vi "rqcBob FPGA.vi"() -> ()   [LabVIEW 2018]
uses:
  rqcBob/Custom Controls/rqcBob Trigger Type.ctl
  rqcBob/Custom Controls/Main State Machine/rqcBob Main SM.ctl
  rqcBob/Custom Controls/Main State Machine/rqcBob Main Operation State.ctl
  rqcBob/Custom Controls/Main State Machine/rqcBob Main Operation Parameters.ctl
  rqcBob/Custom Controls/Pulse Train/rqcBob Pulse Train Config.ctl
  rqcBob/Custom Controls/Pulse Train/rqcBob Pulse Train.Generation Mode.ctl
  rqcBob/Custom Controls/Pulse Train/rqcBob Pulse Train.First Pulse Delay Mode.ctl
  rqcBob/Custom Controls/rqcBob Modulator Config.ctl
  rqcBob/Custom Controls/rqcBob Window Config.ctl
  rqcBob/Custom Controls/rqcBob Detector Settings.ctl
  Shared/Shared FPGA Lib/Shared Logic/Custom Controls/rqc Random Generator.parameters.ctl
  Shared/Shared FPGA Lib/Shared Logic/Custom Controls/rqc Random Generator.value type.ctl
  <vilib>/Platform/TimedLoop/XDataNode/timing_clust.ctl
  <vilib>/Platform/TimedLoop/XDataNode/nitl_modes.ctl
  <vilib>/Platform/TimedLoop/XDataNode/wakeup.ctl
  <vilib>/rvi/Emulation/niFpgaSctlEmulationGetInTimedLoop.vi
  <vilib>/rvi/Emulation/niFpgaEmulationReportErrorSimple.vi
  <vilib>/rvi/Emulation/niFpgaGetClockAttributes.vi
  <vilib>/rvi/Emulation/niFpgaCriticalErrorInLSC.vi
  <vilib>/rvi/eio/common/nirviEmuTemplateMethod_errors.vi
  <vilib>/rvi/Emulation/niFpgaProcessEmulError.vi
  <vilib>/rvi/Emulation/niFpgaEmulationIsFPGAContextNoSignature.vi
  <vilib>/rvi/DataTransferAndStorage/Container/Common/niFpgaContainerGetUniqueNameForEmu.vi
  <vilib>/rvi/Memory/Memory_Emulation/niFpgaMemoryEmulationCacheClearOnFirstRun.vi
  <vilib>/rvi/Memory/Memory_Emulation/nirvimemoryEmulationManagerCache_MakeExclusive.vi
  <vilib>/rvi/Memory/Memory_Emulation/niFpgaMemoryEmulationValidateCache.vi
  <vilib>/rvi/Memory/Memory_Emulation/nirvimemoryEmulationManagerCache_InsertValue.vi
  <vilib>/Utility/error.llb/Clear Errors.vi
  <vilib>/rvi/Memory/Memory_Emulation/nirvimemoryEmulationManagerCache_ReleaseExclusive.vi
  <vilib>/rvi/Memory/Memory_Emulation/nirvimemoryEmulationManagerCache_GetValue.vi
  <vilib>/rvi/Memory/Memory_Emulation/nirvimemoryEmulationManagerCache_SetValue.vi
  <vilib>/rvi/eio/common/nirviEmuReportErrorAndStop.vi
  Shared/Shared FPGA Lib/Shared Logic/FIFO/FIFO.write/rqc FIFO Write (U32).vi
  Shared/Shared FPGA Lib/Shared Logic/FIFO/FIFO.write/rqc FIFO Write (U16).vi
  <vilib>/RQC/FPGA Basic Logic/Counters/Counter (U8).vi
  <vilib>/rvi/DataTransferAndStorage/Container/Common/niFpgaContainerSetEmuInfo.vi
  <vilib>/Platform/TimedLoop/XDataNode/XDataNode.xnode
  <vilib>/eio/EIONode/EIONode.xnode
  <vilib>/rvi/DataTransferAndStorage/Container/XNode/niFpgaContainer.xnode
  <vilib>/rvi/DataTransferAndStorage/Register/Emulation/niFpgaRegisterEmulation.vi
  <vilib>/rvi/DataTransferAndStorage/Handshake/Emulation/niFpgaHandshakeEmulation.vi
  <vilib>/rvi/LocalResourceManager/LocalResourceManager.xnode
  <vilib>/Platform/TimedLoop/XDataNode/XDNodeRunTimeDep.lvlib
panel:
  in  "rndGen.levels values":u16[](array[numeric])=[0, 0, 0, 0]
  in  "rndGen.num of levels":u16
  in  "rndGen.constant":u16
  in  "rndGen.value type":T1=enum."constant"
  out "rndGen.parameters":T2={"value type"=enum."constant", "constant"=0, "num of levels"=0, "levels values"=[0, 0, 0, 0]}
  in  "window.close":u16
  in  "window.open":u16
  in  "modulator.stop":u16
  in  "modulator.start":u16
  in  "train.first pulse delay":u16
  in  "train.first pulse delay mode":T3
  in  "train.num of trains":u16
  in  "train.mode":T4
  in  "train.num of pulses":u16
  in  "train.period":u16
  out "PD.fifo overflow":bool
  in  "rndGen.initial seed":u32=4294967295 caption="seed"
  out "detector config":T5
  in  "modulator.clock delay":fxp<+,4,4>
  out "Main Config":T6
  in  "rndGen.reset":bool caption="reset"
  in  "PD.use window":bool
  out "rqcBob Main State":T10={"state"=enum."ready for trigger", "trains generated"=0, "current period"=0, "pulses generated"=0}
  in  "PD.detect fifo write enable":bool[](array[boolean])=[FALSE, FALSE]
  in  "PD.state fifo write enable":bool
  out "PD.state fifo oferflow":bool
  in  "PD.max meas length":u32
  in  "PD1.detection window":u8
  in  "PD2.detection window":u8
  out "generation.done":bool
  in  "train.software trigger":bool
  in  "train.trigger type":T12=enum."immediate"
  in  "main.initiate":bool
  in  "main.reset":bool
  # "Main Operation"
  # "Random number generator"
  # "train.config"
  # "modulator.config"
  # "window.config"
  # "Photone Detectors"
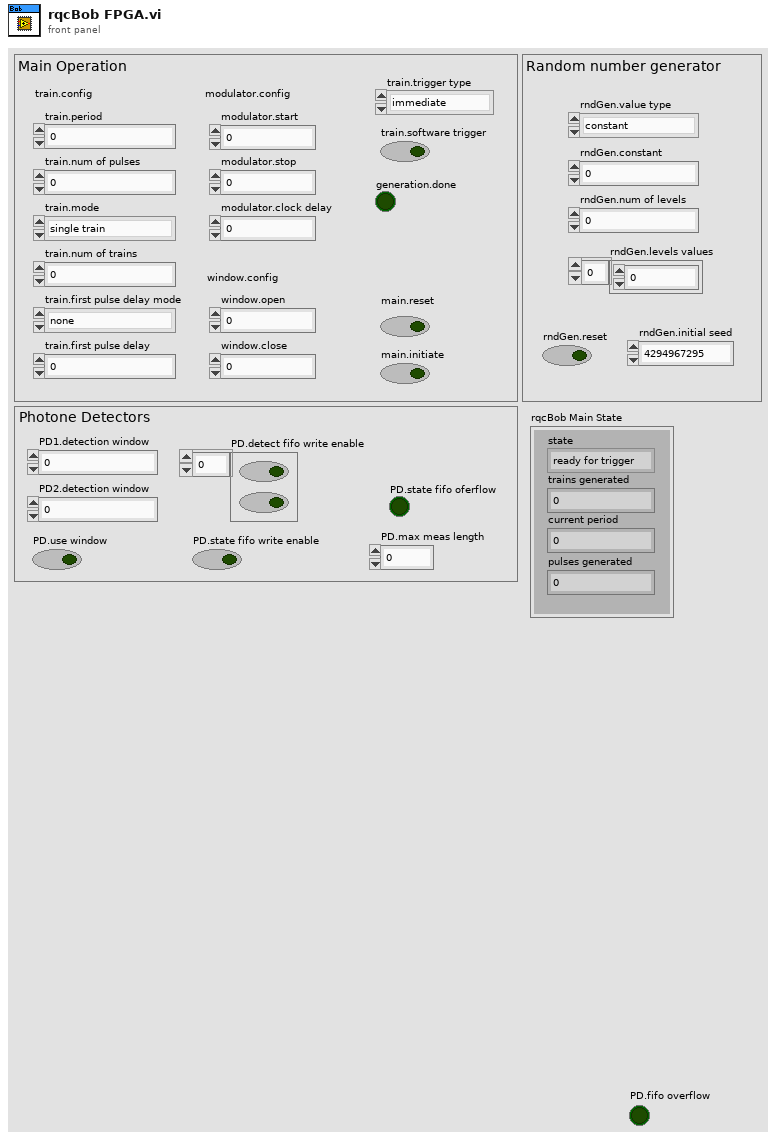
[diagram p1: front panel]
types:
  T1 = typedef "rqc Random Generator.value type.ctl" = enum16{"random value", "constant"}
  T2 = typedef "rqc Random Generator.parameters.ctl" = cluster{"value type":T1, "constant":u16, "num of levels":u16, "levels values":u16[]}
  T3 = typedef "rqcBob Pulse Train.First Pulse Delay Mode.ctl" = enum8{"none", "every train", "first train"}
  T4 = typedef "rqcBob Pulse Train.Generation Mode.ctl" = enum8{"single train", "train sequence.single", "train sequence.wait for trigger", "continuous"}
  T5 = typedef "rqcBob Detector Settings.ctl" = cluster{"PD1.window":u16, "PD2.window":u16, "use window":bool}
  T6 = typedef "rqcBob Main Operation Parameters.ctl" = cluster{"train.configuration":T7, "modulator.config":T8, "window.config":T9}
  T7 = typedef "rqcBob Pulse Train Config.ctl" = cluster{"period":u16, "num of pulses":u16, "mode":T4, "num of trains":u16, "first pulse delay mode":T3, "first pulse delay":u16}
  T8 = typedef "rqcBob Modulator Config.ctl" = cluster{"modulator.start":u16, "modulator.stop":u16}
  T9 = typedef "rqcBob Window Config.ctl" = cluster{"window.open":u16, "window.close":u16}
  T10 = typedef "rqcBob Main SM.ctl" = cluster{"state":T11, "trains generated":u16, "current period":u16, "pulses generated":u16}
  T11 = typedef "rqcBob Main Operation State.ctl" = enum8{"idle", "reset", "ready for trigger", "first puls delay", "generate", "end of train"}
  T12 = typedef "rqcBob Trigger Type.ctl" = enum16{"software", "immediate", "DIO"}
  T13 = typedef "XDNodeRunTimeDep.lvlib/timing_clust.ctl" = cluster{"Expected End [f-1]":u64, "Actual End [f-1]":u64, "Finished Late? [f-1]":bool, "Expected End [i-1]":u64, "Actual End [i-1]":u64, "Finished Late? [i-1]":bool, "Expected Start [i]":u64, "Actual Start [i]":u64, "Expected Start [f]":u64, "Actual Start [f]":u64, "Source Name":string, "Structure Name":string, "Period":i64, "Deadline":i64, "Offset":i64, "Start":i64, "Priority":i32, "Timeout":i32, "Mode":T14, "Wakeup Reason":T15, "Error":errorcluster, "Source Type":string, "Secondary Source Type":string, "Global End Time":u64, "Global Start Time":u64, "Frame Duration":u64, "Iteration Duration":u64, "Assigned CPU":i32, "I/O Scan Engine Mode":u32}
  T14 = typedef "XDNodeRunTimeDep.lvlib/nitl_modes.ctl" = enum32{"No Change", "Process missed periods, maintain original phase", "Discard missed periods, maintain original phase", "Process missed periods, ignore original phase", "Discard missed periods, ignore original phase"}
  T15 = typedef "XDNodeRunTimeDep.lvlib/wakeup.ctl" = enum32{"Normal", "Aborted", "Asynchronous wakeup", "Timing source error", "Timed loop error", "Timeout"}
  T16 = typedef "rqcBob HW Control.ctl" = cluster{"laser":bool, "modulator":bool, "window":bool, "rndGen value":u32, "DAC value":u16, "DAC level":u8, "DAC clock":bool, "PD signal":u8, "PD reset":bool}
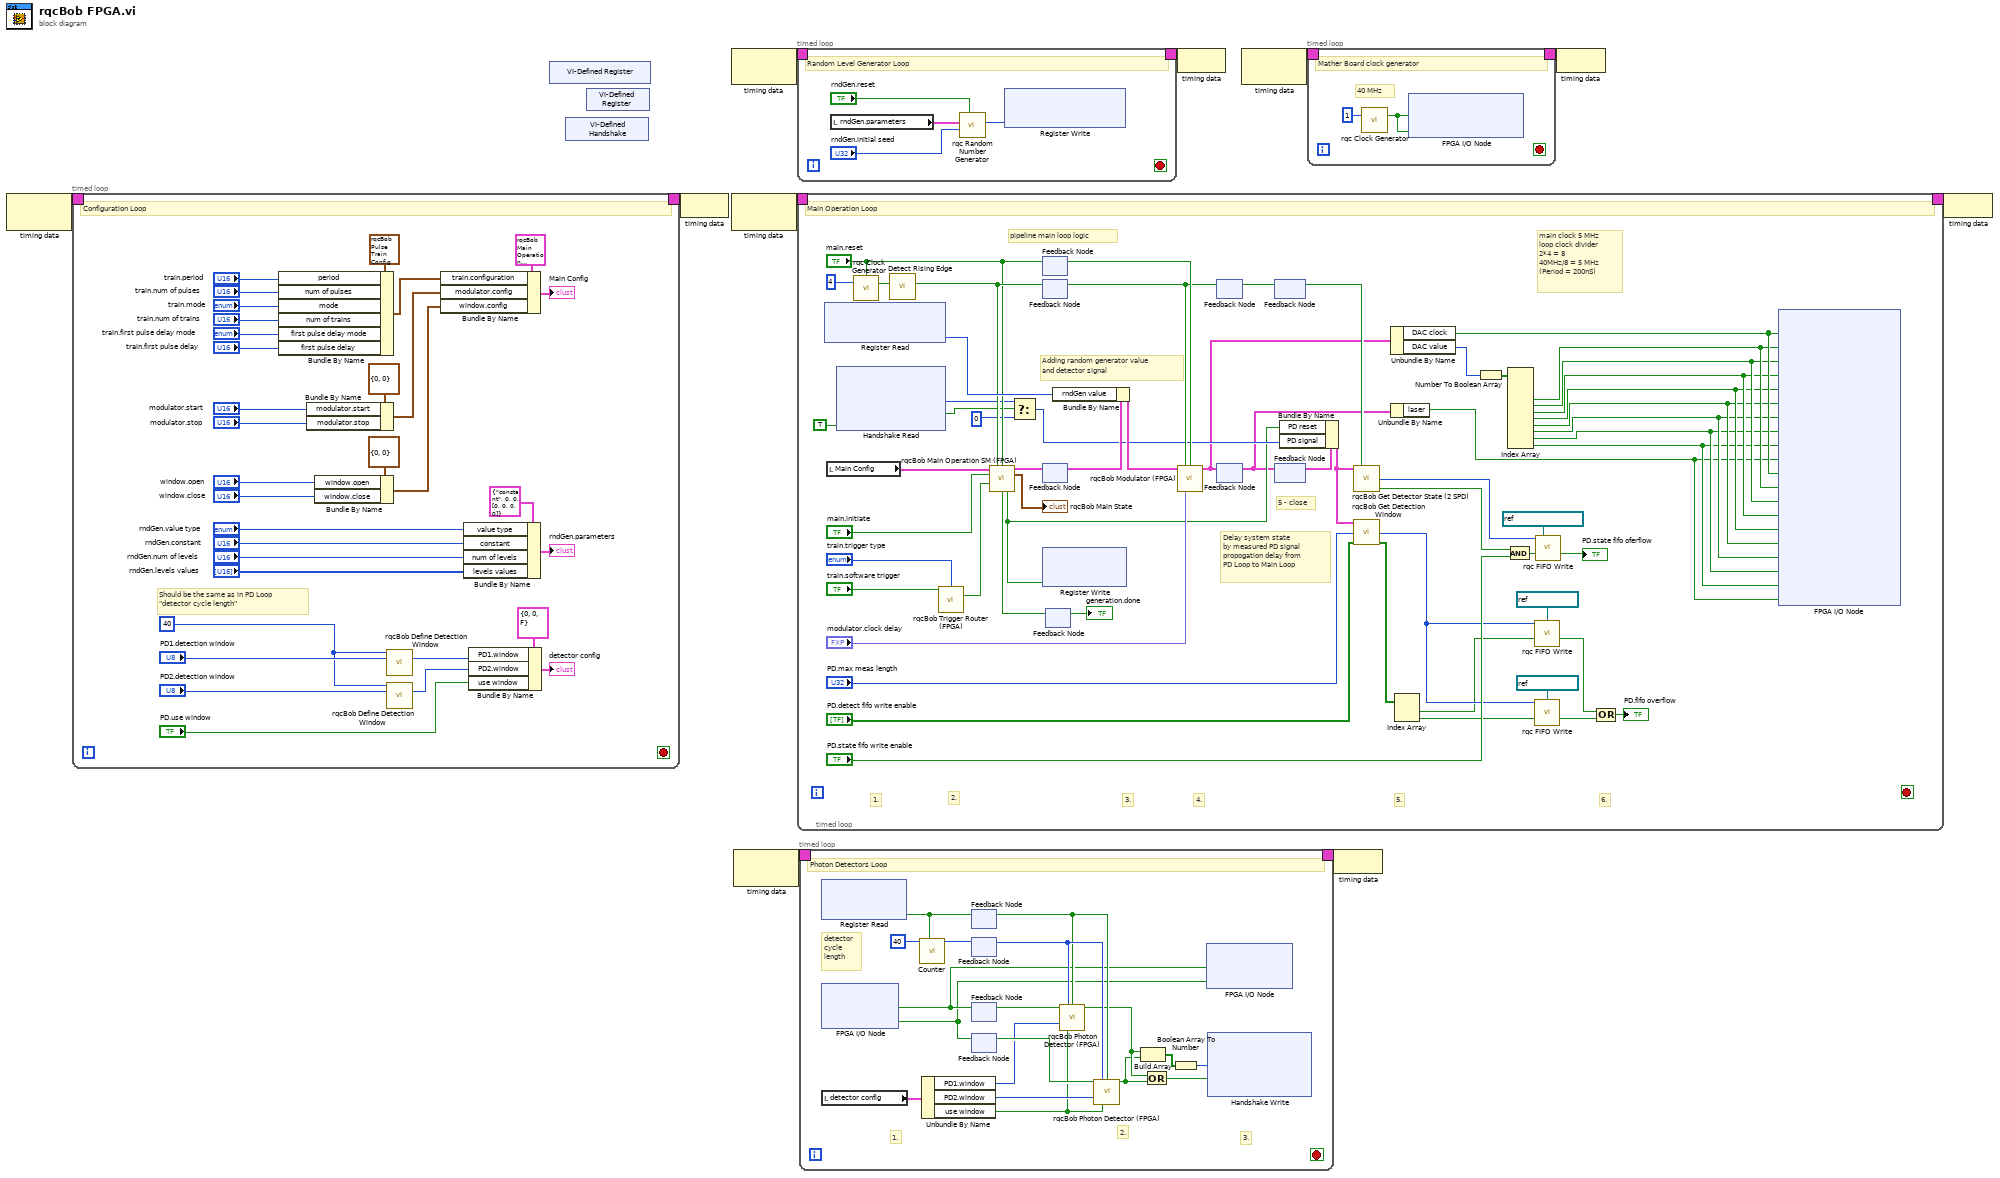
[diagram p0: block diagram]
diagram:
  n1 = node-c288() -> (w2:T13)  [unwired: 1 in]
  n2 = timed-loop {
    timing: w2 -> [_]
    timing-out: [_] -> w1
    stop <- _ stop-if-true
    w39 = u8 40 ("detector.detection cycle length")
    # "Should be the same as in PD Loop\n\"detector cycle length\""
    # "Configuration Loop"
    n3 = Bundle By Name(cluster=T7 {"period"=0, "num of pulses"=0, "mode"=enum."single train", "num of trains"=0, "first pulse delay mode"=enum."none", "first pulse delay"=0} ("train.config"), "period"="train.period", "num of pulses"="train.num of pulses", "mode"="train.mode", "num of trains"="train.num of trains", "first pulse delay mode"="train.first pulse delay mode", "first pulse delay"="train.first pulse delay") -> (w31:T7)
    n4 = Bundle By Name(cluster=T8 {"modulator.start"=0, "modulator.stop"=0} ("modulator.config"), "modulator.start"="modulator.start", "modulator.stop"="modulator.stop") -> (w21:T8)
    n5 = Bundle By Name(cluster=T9 {"window.open"=0, "window.close"=0} ("window.config"), "window.open"="window.open", "window.close"="window.close") -> (w18:T9)
    n6 = call "rqcBob Define Detection Window.vi"("detector.detection cycle length"=w39, "detector.detector window in"="PD1.detection window") -> ("detector.detector window out"=w36:u16)  [unwired: 13 in]
    n7 = call "rqcBob Define Detection Window.vi"("detector.detection cycle length"=w39, "detector.detector window in"="PD2.detection window") -> ("detector.detector window out"=w35:u16)  [unwired: 13 in]
    n8 = Bundle By Name(cluster=T6 {"train.configuration"={"period"=0, "num of pulses"=0, "mode"=enum."single train", "num of trains"=0, "first pulse delay mode"=enum."none", "first pulse delay"=0}, "modulator.config"={"modulator.start"=0, "modulator.stop"=0}, "window.config"={"window.open"=0, "window.close"=0}} ("Main Operation Parameters"), "train.configuration"=w31, "modulator.config"=w21, "window.config"=w18) -> (→"Main Config":T6)
    n9 = Bundle By Name(cluster=T2 {"value type"=enum."constant", "constant"=0, "num of levels"=0, "levels values"=[0, 0, 0, 0]} ("rndGen.parameters"), "value type"="rndGen.value type", "constant"="rndGen.constant", "num of levels"="rndGen.num of levels", "levels values"="rndGen.levels values") -> (→"rndGen.parameters":T2)
    n10 = Bundle By Name(cluster=T5 {"PD1.window"=0, "PD2.window"=0, "use window"=FALSE} ("detector settings"), "PD1.window"=w36, "PD2.window"=w35, "use window"="PD.use window") -> (→"detector config":T5)
  }
  n11 = xnode "VI-Defined Register"() -> ()  [unwired: 1 out]
  n12 = xnode "VI-Defined Handshake"() -> ()  [unwired: 1 out]
  n13 = xnode "VI-Defined Register"() -> ()  [unwired: 1 out]
  n14 = node-c288(w1) -> ()
  n15 = node-c288() -> (w4:T13)  [unwired: 1 in]
  n16 = node-c288() -> (w8:T13)  [unwired: 1 in]
  n17 = node-c288() -> (w6:T13)  [unwired: 1 in]
  n18 = timed-loop {
    timing: w4 -> [_]
    timing-out: [_] -> w3
    stop <- _ stop-if-true
    # "Random Level Generator Loop"
    n19 = local read "rndGen.parameters"() -> (w45:T2)
    n20 = call "rqc Random Number Generator.vi"("reset"="rndGen.reset", "initial seed"="rndGen.initial seed", "rndGen.parameters"=w45) -> ("DAC random value"=w47:u32)  [unwired: 8 in]
    n21 = xnode ("Register Write")("Data"=w47) -> ()  [unwired: 1 in, 1 out]
  }
  n22 = timed-loop {
    timing: w8 -> [_]
    timing-out: [_] -> w7
    stop <- _ stop-if-true
    # "5 - close"
    # "Delay system state\nby measured PD signal\npropogation delay from \nPD Loop to Main Loop"
    # "Adding random generator value\nand detector signal"
    # "main clock 5 MHz\nloop clock divider\n2*4 = 8\n40MHz/8 = 5 MHz \n(Period = 200nS)"
    # "6."
    # "5."
    # "4."
    # "3."
    # "2."
    # "1."
    # "pipeline main loop logic"
    # "Main Operation Loop"
    n23 = xnode ("Register Read")() -> ("Data"=w96:u32)  [unwired: 1 in, 1 out]
    n24 = local read "Main Config"() -> (w101:T6)
    n25 = xnode ("Handshake Read")("Ready for Output"=TRUE) -> ("Data"=w71:u8, "Output Valid"=w72:bool)  [unwired: 1 in, 1 out]
    n26 = call "rqc Clock Generator.vi"("reset"="main.reset", "SCTL clock devider"=u8 4 ("bound")) -> ("clock out"=w88:bool)  [unwired: 13 in]
    n27 = call <vilib>:"Detect Rising Edge.vi"("signal"=w88) -> ("edge detected"=w87:bool)  [unwired: 10 in]
    n28 = call "rqcBob Trigger Router (FPGA).vi"("sw"="train.software trigger", "rqcBob Trigger Type"="train.trigger type") -> ("trigger out"=w109:bool)  [unwired: 13 in]
    n29 = call "rqcBob Main Operation SM (FPGA).vi"("Main Operation Parameters"=w101, "clock in"=w87, "reset"="main.reset", "initiate"="main.initiate", "trigger"=w109) -> ("HW state"=w85:T16, "rqcBob Main State"=→"rqcBob Main State":T10, "done"=w102:bool, "detector.reset"=w64:bool)  [unwired: 7 in]
    n30 = Select(t=w71, s=w72, f=u8 0) -> (s? t:f=w65:u8)
    n31 = feedback #1() -> (w100:bool)  [unwired: 1 in]
    n32 = feedback-in #1("main.reset") -> ()
    n33 = feedback #2() -> (w68:bool)  [unwired: 1 in]
    n34 = feedback-in #2(w87) -> ()
    n35 = feedback #3() -> (w98:T16)  [unwired: 1 in]
    n36 = feedback-in #3(w85) -> ()
    n37 = xnode ("Register Write")("Data"=w64) -> ()  [unwired: 1 in, 1 out]
    n38 = feedback #4() -> (→"generation.done":bool)  [unwired: 1 in]
    n39 = feedback-in #4(w102) -> ()
    n40 = Bundle By Name(cluster=w98, "rndGen value"=w96) -> (w97:T16)
    n41 = call "rqcBob Modulator (FPGA).vi"("rqcBob HW Control in"=w97, "clock in"=w68, "reset"=w100, "mod.clock delay"="modulator.clock delay") -> ("rqcBob HW Control out"=w62:T16)  [unwired: 11 in]
    n42 = feedback-in #5(w68) -> ()
    n43 = feedback #5() -> (w63:bool)  [unwired: 1 in]
    n44 = feedback-in #6(w62) -> ()
    n45 = feedback #6() -> (w61:T16)  [unwired: 1 in]
    n46 = feedback #7() -> (w67:bool)  [unwired: 1 in]
    n47 = feedback-in #7(w63) -> ()
    n48 = feedback-in #8(w61) -> ()
    n49 = feedback #8() -> (w69:T16)  [unwired: 1 in]
    n50 = Bundle By Name(cluster=w69, "PD reset"=w64, "PD signal"=w65) -> (w66:T16)
    n51 = call "rqcBob Get Detector State (2 SPD).vi"("rqcBob HW Control in"=w66, "clock in"=w67) -> ("SPD state"=w92:u16, "write to fifo"=w93:bool)  [unwired: 11 in, 1 out]
    n52 = call "rqcBob Get Detection Window.vi"("rqcBob HW Control in"=w66, "PD.max meas length"="PD.max meas length", "PD.detect fifo write enable"="PD.detect fifo write enable") -> ("window"=w77:u32, "PD clicked"=w76:bool[])  [unwired: 10 in, 1 out]
    n53 = Unbundle By Name(w62) -> ("DAC clock"=w60:bool, "DAC value"=w94:u16)
    n54 = Unbundle By Name(w61) -> ("laser"=w51:bool)
    n55 = Index Array(array=w76) -> (element #1=w75:bool, element #2=w74:bool)  [unwired: 2 in]
    n56 = Number To Boolean Array(number=w94) -> (Boolean array=w106:bool[])
    n57 = Index Array(array=w106) -> (element #3=w59:bool, element #4=w58:bool, element #5=w57:bool, element #6=w56:bool, element #7=w55:bool, element #8=w54:bool, element #9=w53:bool, element #10=w52:bool)  [unwired: 10 in, 2 out]
    n58 = Compound Arithmetic op=AND(w93, "PD.state fifo write enable") -> (w91:bool)
    n59 = call-poly "rqc FIFO Write.vi"("Element"=w77, "FIFO"=refnum<k21> "FIFO PD1" ("FIFO SPD"), "data valid"=w75) -> ("fifo overflow"=w79:bool)  [unwired: 12 in]
    n60 = call-poly "rqc FIFO Write.vi"("Element"=w77, "FIFO"=refnum<k21> "FIFO PD2" ("FIFO SPD"), "data valid"=w74) -> ("fifo overflow"=w78:bool)  [unwired: 12 in]
    n61 = call-poly "rqc FIFO Write.vi"("Element"=w92, "FIFO"=refnum<k21> "FIFO PD State" ("FIFO In"), "data valid"=w91) -> ("SPD.state fifo oferflow"=→"PD.state fifo oferflow":bool)  [unwired: 12 in]
    n62 = Compound Arithmetic op=OR(w79, w78) -> (→"PD.fifo overflow":bool)
    n63 = xnode "FPGA I/O Node"("DAC/clock"=w60, "DAC/bit2"=w59, "DAC/bit3"=w58, "DAC/bit4"=w57, "DAC/bit5"=w56, "DAC/bit6"=w55, "DAC/bit7"=w54, "DAC/bit8"=w53, "DAC/bit9"=w52, "Laser"=w51, "DAC/clock (service)"=w60, "DAC/bit2 (service)"=w59, "DAC/bit3 (service)"=w58, "DAC/bit4 (service)"=w57, "DAC/bit5 (service)"=w56, "DAC/bit6 (service)"=w55, "DAC/bit7 (service)"=w54, "DAC/bit8 (service)"=w53, "DAC/bit9 (service)"=w52, "Laser (service)"=w51) -> ()  [unwired: 20 in, 20 out]
  }
  n64 = timed-loop {
    timing: w6 -> [_]
    timing-out: [_] -> w5
    stop <- _ stop-if-true
    # "detector\ncycle \nlength"
    # "3."
    # "2."
    # "1."
    # "Photon Detectors Loop"
    n65 = xnode ("Register Read")() -> ("Data"=w115:bool)  [unwired: 1 in, 1 out]
    n66 = xnode "FPGA I/O Node"() -> ("D1 Signal"=w114:bool, "D2 Signal"=w113:bool)  [unwired: 2 in, 2 out]
    n67 = local read "detector config"() -> (w125:T5)
    n68 = call-poly <vilib>:"Counter.vi"("reset"=w115, "bound"=u8 40 ("SPD.detection cycle length")) -> ("count out"=w130:u8)  [unwired: 8 in, 1 out]
    n69 = Unbundle By Name(w125) -> ("PD1.window"=w124:u16, "PD2.window"=w123:u16, "use window"=w121:bool)
    n70 = feedback-in #9(w115) -> ()
    n71 = feedback #9() -> (w122:bool)  [unwired: 1 in]
    n72 = feedback #10() -> (w129:u8)  [unwired: 1 in]
    n73 = feedback-in #10(w130) -> ()
    n74 = feedback #11() -> (w128:bool)  [unwired: 1 in]
    n75 = feedback-in #11(w114) -> ()
    n76 = feedback #12() -> (w127:bool)  [unwired: 1 in]
    n77 = feedback-in #12(w113) -> ()
    n78 = call "rqcBob Photon Detector (FPGA).vi"("detector signal in"=w128, "current cycle"=w129, "reset"=w122, "detector.detector window"=w124, "detector.use detector window"=w121) -> ("detector out"=w118:bool)  [unwired: 10 in]
    n79 = call "rqcBob Photon Detector (FPGA).vi"("detector signal in"=w127, "current cycle"=w129, "reset"=w122, "detector.detector window"=w123, "detector.use detector window"=w121) -> ("detector out"=w117:bool)  [unwired: 10 in]
    n80 = Build Array(w118, w117) -> (w119:bool[])
    n81 = Compound Arithmetic op=OR(w118, w117) -> (w116:bool)
    n82 = Boolean Array To Number(Boolean array=w119) -> (number=w120:u8)
    n83 = xnode "FPGA I/O Node"("D1 (service)"=w114, "D2 (service)"=w113) -> ()  [unwired: 2 in, 2 out]
    n84 = xnode ("Handshake Write")("Data"=w120, "Input Valid"=w116) -> ()  [unwired: 1 in, 2 out]
  }
  n85 = node-c288(w3) -> ()
  n86 = node-c288() -> (w10:T13)  [unwired: 1 in]
  n87 = timed-loop {
    timing: w10 -> [_]
    timing-out: [_] -> w9
    stop <- _ stop-if-true
    # "40 MHz"
    # "Mather Board clock generator"
    n88 = call "rqc Clock Generator.vi"("SCTL clock devider"=u8 1 ("MBClock.80M clock devider")) -> ("clock out"=w133:bool)  [unwired: 14 in]
    n89 = xnode "FPGA I/O Node"("MBClock"=w133, "MBClock (service)"=w133) -> ()  [unwired: 2 in, 2 out]
  }
  n90 = node-c288(w5) -> ()
  n91 = node-c288(w9) -> ()
  n92 = node-c288(w7) -> ()
